vi "TC_Calibrate_Multi.vi"(7 "TC_Type_Array":T1[](array[typedef])=[3, 3, 3, 3, 3, 3, 3, 3, 3, 3, 3, 3, 3, 3, 3, 3] items=["B", "E", "J", "K", "R", "S", "T", "N"], 10 "TC in":dbl[](array[numeric])) -> (2 "TC out":sgl[](array[numeric]))   [LabVIEW 2014]
uses:
  Program Files (x86)/National Instruments/LabVIEW 2014/examples/CompactRIO/Shared/cRIO Convert Thermocouple Readings.llb/Thermocouple Type.ctl
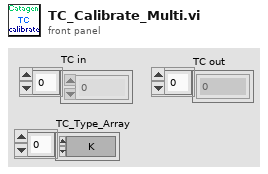
[diagram p1: front panel]
types:
  T1 = typedef "Thermocouple Type.ctl" = u16
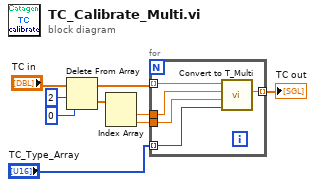
[diagram p0: block diagram]
diagram:
  n1 = Delete From Array(array="TC in", length=2, index=0) -> (deleted portion=w5:dbl[], array with subset deleted=w6:dbl[])
  n2 = Index Array(array=w5) -> (element #1=w4:dbl, element #2=w3:dbl)  [unwired: 2 in]
  n3 = for {
    tunnel: w3 -> [w12]
    tunnel: w4 -> [w13]
    tunnel: w6 -> [w14] mode=indexing
    tunnel: [w10] -> w2 mode=indexing
    tunnel: "TC_Type_Array" -> [w11] mode=indexing
    n4 = call "Convert to T_Multi.vi"("ThermocoupleType"=w11, "CJC"=w12, "AutoZero"=w13, "TC Input"=w14) -> ("Linearized Temperature"=w10:sgl)  [unwired: 7 in]
  }
  "TC out" <- w2
